vi "FindRobotByRole_v2.vi"(8 "error in (no error)":errorcluster, 9 "role":T1=enum."DefenderArea", 10 "Array":refnum<class "Robot.lvclass">[](array[class]), 11 "object in":refnum<class "Utilities.lvclass">) -> (0 "error out":errorcluster, 1 "foundRobot":bool, 2 "Robot":refnum<class "Robot.lvclass">, 3 "object out":refnum<class "Utilities.lvclass">)   [LabVIEW 2023, in "Utilities.lvclass"]
uses:
  Utilities.lvclass
  Utilities.lvclass/Utilities.ctl
  Robot_class/Robot.lvclass
  Robot_class/roles.ctl
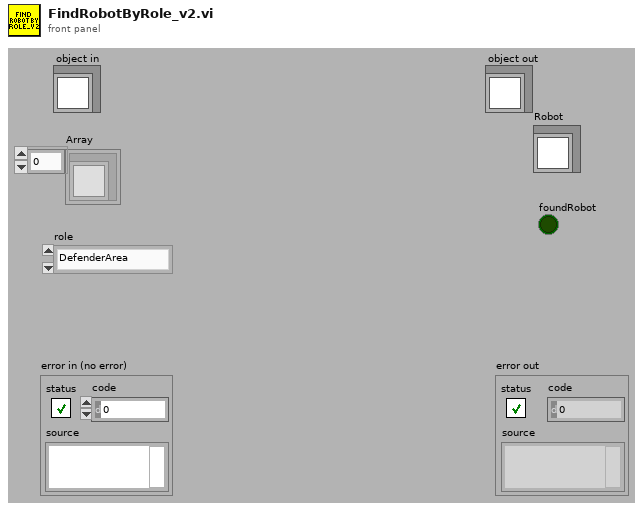
[diagram p1: front panel]
types:
  T1 = typedef "roles.ctl" = enum16{"SimpleBallPlacement", "BallPlacementAllyPasser", "BallPlacementAllyReceiver", "BallPlacementEnemy", "5Robots5th", "PassBestReceiver", "5Robots4th", "5Robots3rd", "5Robots2nd", "5Robots1st", "PassBestRobot", "WaitPass", "ABCThirdKicker", "ABCFirstKicker", "ABCSecondKicker", "Tabler", "TableFinalizer", "PrepareRollToPassRoller", "PrepareRollToPassReceiver", "SimplePassRoll", "SimplePassRollReceiver", "PenaltyDefense", "PreparePassReceiver 2", "PreparePassReceiver 1", "PassObserver", "Timeout", "Goto", "ZigZag", "None", "BallOutOfField", "DefenderArea", "Duelist", "AttackerStop", "FollowAttacker", "KeeperRole", "KickPenalty", "AttackerAimGoal", "AttackerBlock", "Marker", "Halt", "Shoot", "PassKicker", "PassReceiver", "TestRole", "PenaltyAttacker", "PrimaryAttackerRole", "SupportAttackerRole"}
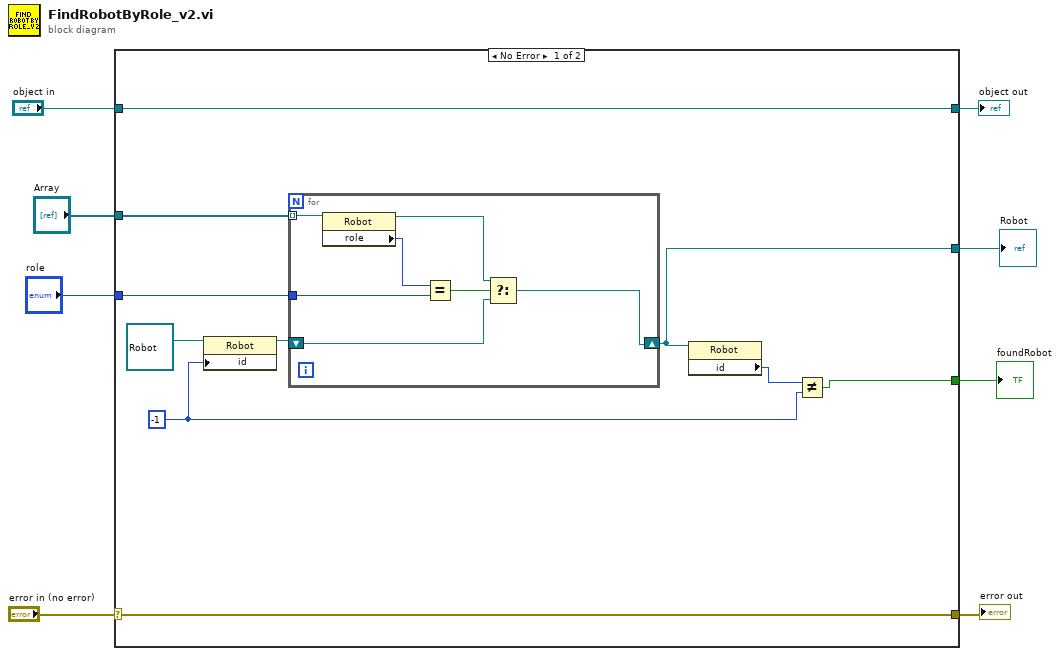
[diagram p0: block diagram]
diagram:
  n1 = case shown="No Error" "error in (no error)" {
    selector: "error in (no error)" -> [w18 w27]
    tunnel: [w18 w27] -> w7
    tunnel: [w17 w26] -> w5
    tunnel: "object in" -> [w17 w26]
    tunnel: "Array" -> [w16 _]
    tunnel: "role" -> [w15 _]
    tunnel: [w14 _] -> w2
    tunnel: [w9 _] -> w1
    frame No Error {
      w10 = -1 ("id")
      n2 = property class="Robot"(reference=refnum<class "Robot.lvclass"> refnum ("Robot"), "id"=w10) -> (reference out=w12:refnum<class "Robot.lvclass">)  [unwired: 1 in, 1 out]
      n3 = for {
        tunnel: w16 -> [w25] mode=indexing
        tunnel: w15 -> [w23]
        shift-right: [w19] -> w14
        shift-left: w12 -> [w21]
        n4 = property class="Robot"(reference=w25) -> (reference out=w20:refnum<class "Robot.lvclass">, "role"=w24:T1)  [unwired: 1 in, 1 out]
        n5 = Equal?(x=w24, y=w23) -> (x = y?=w22:bool)
        n6 = Select(t=w20, s=w22, f=w21) -> (s? t:f=w19:refnum<class "Robot.lvclass">)
      }
      n7 = property class="Robot"(reference=w14) -> ("id"=w11:i32)  [unwired: 1 in, 2 out]
      n8 = Not Equal?(x=w11, y=w10) -> (x != y?=w9:bool)
    }
    frame Error {
    }
  }
  "error out" <- w7
  "object out" <- w5
  "Robot" <- w2
  "foundRobot" <- w1
